vi "From Variant.vi"(8 "Error In":errorcluster, 10 "Variant":variant, 11 "TD Int A In":refnum<class "1D Int.lvclass">) -> (0 "Error Out":errorcluster, 3 "TD Int A Out":refnum<class "1D Int.lvclass">)   [LabVIEW 2017, in "Tree API.lvlib" / "1D Int.lvclass"]
doc: "Dynamic dispatch interface for conversion of variant LV data to Tree Data classes."
uses:
  1D Int.lvclass
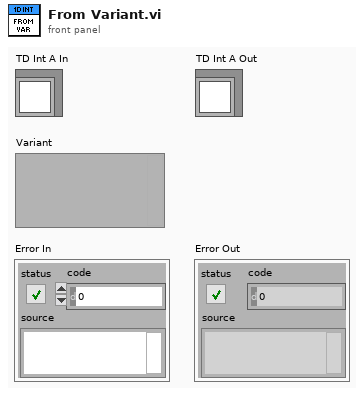
[diagram p1: front panel]
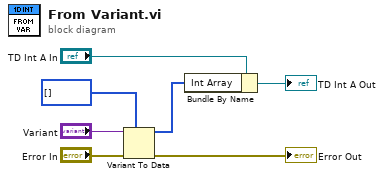
[diagram p0: block diagram]
diagram:
  n1 = Variant To Data(error in="Error In", type=i64[] [] ("Int Array"), Variant="Variant") -> (data=w2:i64[], error out=→"Error Out":errorcluster)
  n2 = Bundle By Name(cluster="TD Int A In", "Int Array"=w2) -> (→"TD Int A Out":refnum<class "1D Int.lvclass">)
